vi "LCOS Pattern Display_green.vi"() -> ()   [LabVIEW 2011]
uses:
  <vilib>/Utility/miscctls.llb/LVRectTypeDef.ctl
  LCOS Pattern Display Actions.ctl
  <vilib>/vision/Image Controls.llb/IMAQ Image.ctl
panel:
  out "Image":T1(plugin-control)
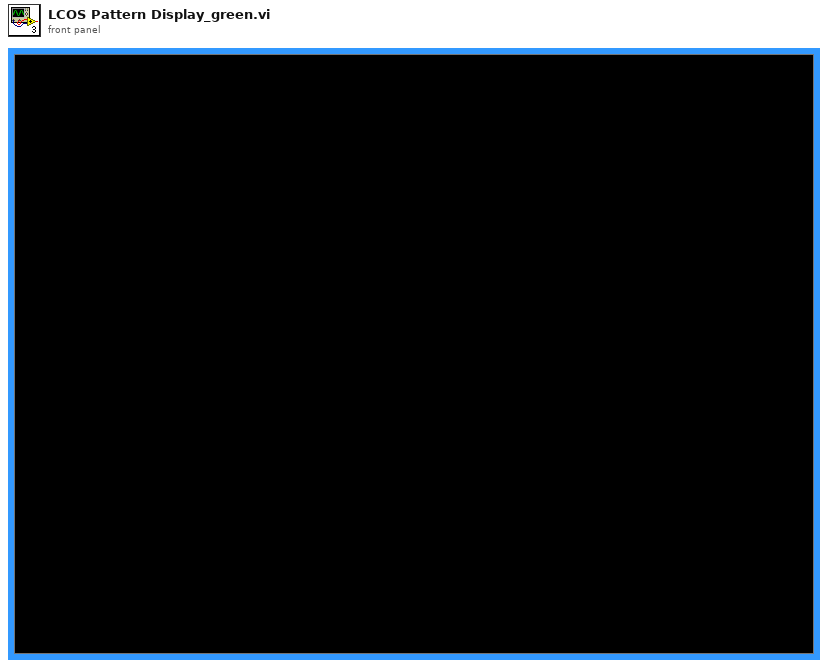
[diagram p1: front panel]
types:
  T1 = typedef "IMAQ Image.ctl" = refnum<image>
  T2 = typedef "LCOS Pattern Display Actions.ctl" = enum16{"Init", "Idle", "Update", "Exit"}
  T3 = cluster{"LCOS Pattern Display Actions":T2, "Data":variant}
  T4 = typedef "LVRectTypeDef.ctl" = cluster{"Left":i16, "Top":i16, "Right":i16, "Bottom":i16}
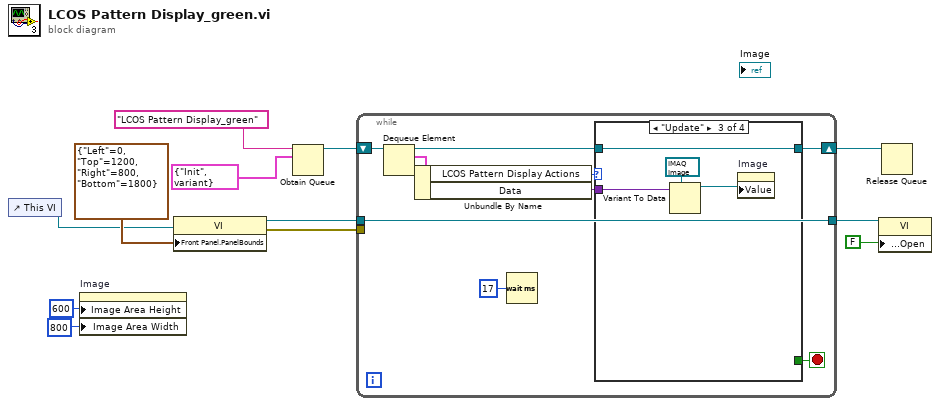
[diagram p0: block diagram]
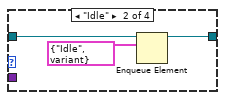
[diagram p3: hidden frame]
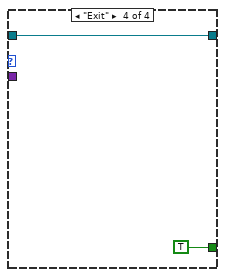
[diagram p4: hidden frame]
diagram:
  n1 = control-ref of="This VI"() -> (w1:refnum<vi>)
  n2 = property on="Image" class="ImageControl"("Image Area Height"=u32 600 ("Image Area:Size:Height"), "Image Area Width"=u32 800 ("y")) -> ()  [unwired: 2 in, 2 out]
  n3 = property class="VI"(reference=w1, "Front Panel.PanelBounds"=T4 {"Left"=0, "Top"=1200, "Right"=800, "Bottom"=1800} ("Front Panel Window:Panel Bounds")) -> (reference out=w6:refnum<vi>, error out=w10:errorcluster)  [unwired: 1 in]
  n4 = Obtain Queue(name (unnamed)="LCOS Pattern Display_green", element data type=T3 {"LCOS Pattern Display Actions"=enum."Init", "Data"=variant}) -> (queue out=w8:refnum<queue>)  [unwired: 3 in, 2 out]
  n5 = while {
    tunnel: w10 -> [_]
    shift-right: [w16] -> w3
    shift-left: w8 -> [w21]
    tunnel: w6 -> [w15]
    tunnel: [w15] -> w4
    stop <- w18 stop-if-true
    n6 = Dequeue Element(queue=w21) -> (queue out=w17:refnum<queue>, element=w20:T3)  [unwired: 2 in, 2 out]
    n7 = Unbundle By Name(w20) -> ("LCOS Pattern Display Actions"=w19:T2, "Data"=w13:variant)
    n8 = Wait (ms)(milliseconds to wait=u32 17) -> ()  [unwired: 1 out]
    n9 = case shown="\"Update\"" w19 {
      tunnel: [_ _ _ TRUE] -> w18
      tunnel: w17 -> [w22 w25 w27 w30]
      tunnel: [w22 w24 w27 w30] -> w16
      tunnel: w13 -> [_ _ w29 _]
      frame "Init", Default {
      }
      frame "Idle" {
        n10 = Enqueue Element(queue=w25, element=T3 {"LCOS Pattern Display Actions"=enum."Idle", "Data"=variant}) -> (queue out=w24:refnum<queue>)  [unwired: 2 in, 2 out]
      }
      frame "Update" {
        n11 = Variant To Data(type=T1 refnum ("Image"), Variant=w29) -> (data=w26:T1)  [unwired: 1 in, 1 out]
        n12 = property on="Image" class="ImageControl"("Value"=w26) -> ()  [unwired: 2 in, 2 out]
      }
      frame "Exit" {
      }
    }
  }
  n13 = property class="VI"(reference=w4, "Front Panel.Open"=FALSE ("Front Panel Window:Open")) -> ()  [unwired: 1 in, 2 out]
  n14 = Release Queue(queue=w3) -> ()  [unwired: 2 in, 3 out]
